vi "Load Plugins.vi"(8 "error in (no error)":errorcluster, 11 "PlatformManager in":refnum<class "PlatformManager.lvclass">) -> (0 "error out":errorcluster, 3 "PlatformManager out":refnum<class "PlatformManager.lvclass">)   [LabVIEW 2020, in "PicoG-Core.lvlib" / "PlatformManager.lvclass"]
uses:
  PlatformManager.lvclass
  PlatformManager.lvclass/PlatformManager.ctl
  Platform/Platform.lvclass
  <vilib>/Utility/LVLibp/NI_PackedLibraryUtility.lvlib
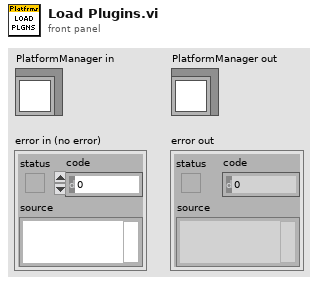
[diagram p1: front panel]
types:
  T1 = typedef "PicoG-Core.lvlib/PlatformManager.lvclass/Ref Data.ctl" = cluster{"Platforms":refnum<class "Platform.lvclass">[]}
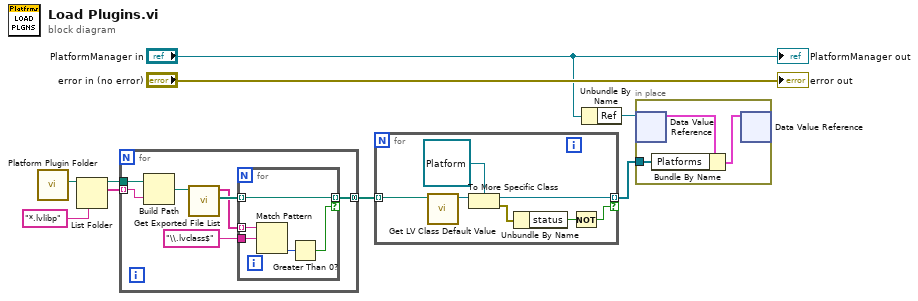
[diagram p0: block diagram]
diagram:
  n1 = call "Platform Plugin Folder.vi"() -> ("Path"=w4:path)  [unwired: 11 in]
  n2 = List Folder(path=w4, pattern="*.lvlibp") -> (path out=w7:path, filenames=w6:string[])  [unwired: 2 in, 2 out]
  n3 = for {
    tunnel: w7 -> [w16]
    tunnel: w6 -> [w15] mode=indexing
    tunnel: [w10] -> w5 mode=concatenating
    n4 = Build Path(base path=w16, name or relative path=w15) -> (appended path=w14:path)
    n5 = call <vilib>:"Get Exported File List.vi"("packed library path"=w14) -> ("paths"=w13:path[], "qualified names"=w12:string[])  [unwired: 8 in, 1 out]
    n6 = for {
      tunnel: w13 -> [w19] mode=indexing
      tunnel: w12 -> [w21] mode=indexing
      tunnel: "\\.lvclass$" ("regular expression") -> [w20]
      tunnel: [w19] -> w10 mode=indexing if=w17
      n7 = Match Pattern(string=w21, regular expression=w20) -> (offset past match=w18:i32)  [unwired: 1 in, 3 out]
      n8 = Greater Than 0?(x=w18) -> (x > 0?=w17:bool)
    }
  }
  n9 = for {
    tunnel: w5 -> [w22] mode=indexing
    tunnel: [w27] -> w1 mode=indexing if=w24
    n10 = call <vilib>:"Get LV Class Default Value.vi"("class path"=w22) -> ("object"=w23:refnum<class>)  [unwired: 9 in, 1 out]
    n11 = To More Specific Class(target class=refnum<class "Platform.lvclass"> refnum ("PicoG-Core:DeployTarget"), reference=w23) -> (specific class reference=w27:refnum<class "Platform.lvclass">, error out=w26:errorcluster)  [unwired: 1 in]
    n12 = Unbundle By Name(w26) -> ("status"=w25:bool)
    n13 = Not(x=w25) -> (.not. x?=w24:bool)
  }
  n14 = Unbundle By Name("PlatformManager in") -> ("Ref"=w3:refnum<data-value>)
  n15 = in-place {
    in-place-border: w1 -> [w29]
    n16 = in-place-dvr #1(w3) -> (w31:T1)  [unwired: 1 out]
    n17 = Bundle By Name(cluster=w31, "Platforms"=w29) -> (w30:T1)
    n18 = in-place-dvr #1(w30) -> ()  [unwired: 2 out]
  }
  "error out" <- "error in (no error)"
  "PlatformManager out" <- "PlatformManager in"
